vi "Analog_to_14bit.vi"(11 "Pockels (0-2V)":dbl) -> (3 "Pockels Level(14 bit)":dbl)   [LabVIEW 2020]
panel:
  in  "numbits":i16=14
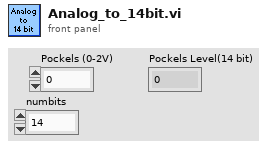
[diagram p1: front panel]
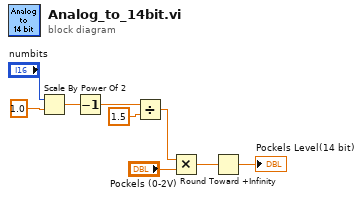
[diagram p0: block diagram]
diagram:
  n1 = Scale By Power Of 2(n="numbits", x=1.0) -> (x*2^n=w3:dbl)
  n2 = Decrement(x=w3) -> (x-1=w7:dbl)
  n3 = Divide(x=w7, y=1.5) -> (x/y=w5:dbl)
  n4 = Multiply(x=w5, y="Pockels (0-2V)") -> (x*y=w6:dbl)
  n5 = Round Toward +Infinity(x=w6) -> (ceil(x): smallest int >= x=→"Pockels Level(14 bit)":dbl)
